vi "HandeEvents.vi"(0 "reference in":refnum<class "Logger.lvclass">, 11 "error in (no error)":errorcluster) -> (4 "reference out":refnum<class "Logger.lvclass">, 14 "dt":u32, 15 "error out":errorcluster)   [LabVIEW 2019, in "Logger.lvclass"]
uses:
  Logger.lvclass
  EventData.ctl
  EventCode.ctl
  Priority.ctl
  Logger.lvclass/Logger.ctl
  2f3f98d4-cfb0-4f81-b92a-0d178dd61f1e.vi
  1c0d0c3d-5d6b-42fa-8895-123650284108.vi
  DatabaseInterface_class/DatabaseInterface.lvclass
panel:
  out "remaining elements":T1[](array[typedef])
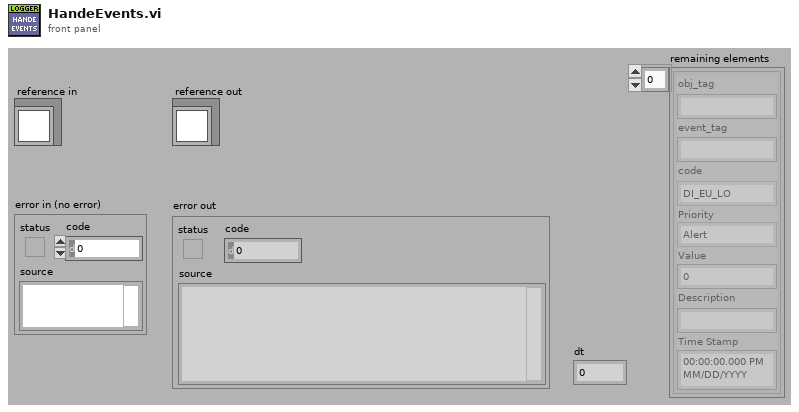
[diagram p1: front panel]
types:
  T1 = typedef "Logger.lvclass/EventData.ctl" = cluster{"obj_tag":string, "event_tag":string, "code":T2, "Priority":T3, "Value":dbl, "Description":string, "Time Stamp":timestamp}
  T2 = typedef "Logger.lvclass/EventCode.ctl" = enum16{"DI_EU_LO", "DI_EU_HI", "DIO_LO", "DIO_HI", "DI_RAW_LO", "DI_RAW_HI", "DO_LO", "DO_HI", "DA_OK", "DA_ALARM", "AA_HI", "AA_HIHI", "AA_LO", "AA_LOLO", "AA_OK", "CMD", "OUT_OF_RANGE_OK", "OUT_OF_RANGE_LO", "OUT_OF_RANGE_HI", "CONFIG", "DI_LO", "DI_HI"}
  T3 = typedef "Logger.lvclass/Priority.ctl" = enum16{"Alert", "Critical", "Error", "Warning", "Notice", "Informational", "Debug"}
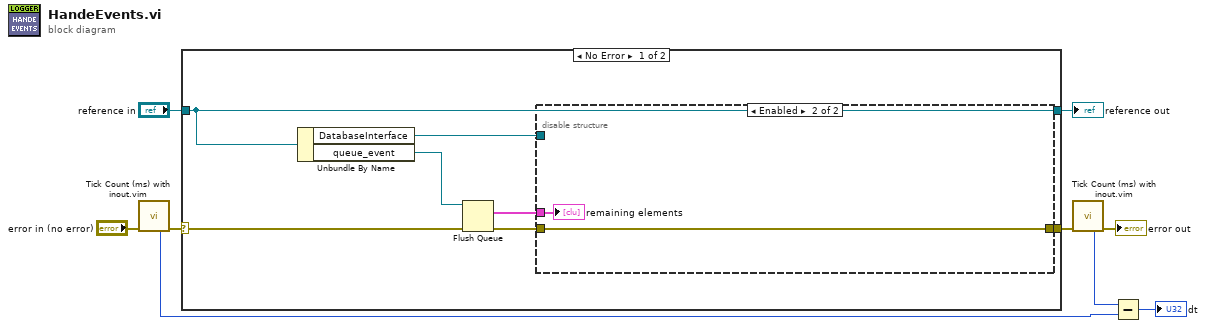
[diagram p0: block diagram]
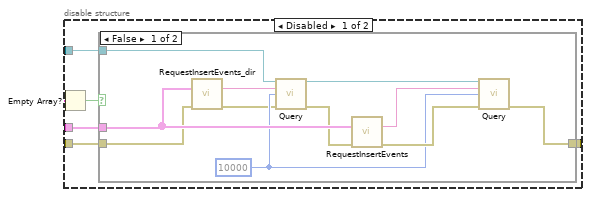
[diagram p2: hidden frame]
diagram:
  n1 = call "Tick Count (ms) with inout.vim"("in"="error in (no error)") -> ("millisecond timer value dub"=w4:u32, "out"=w7:errorcluster)  [unwired: 12 in, 1 out]
  n2 = case shown="No Error" w7 {
    selector: w7 -> [w16 w36]
    tunnel: [w15 w37] -> w2
    tunnel: "reference in" -> [w15 w37]
    tunnel: [w13 w36] -> w1
    frame No Error {
      n3 = Unbundle By Name(w15) -> ("DatabaseInterface"=w11:refnum<class "DatabaseInterface.lvclass">, "queue_event"=w14:refnum<queue>)
      n4 = Flush Queue(queue=w14, error in (no error)=w16) -> (remaining elements=w10:T1[], error out=w12:errorcluster)  [unwired: 1 out]
      n5 = disable-structure shown="Enabled" {
        disable-tunnel: [w21 w34] -> w13
        disable-tunnel: w12 -> [w20 w34]
        disable-tunnel: w11 -> [w19 _]
        disable-tunnel: w10 -> [w18 w35]
        frame Disabled {
          n6 = Empty Array?(array=w18) -> (empty?=w17:bool)
          n7 = case shown="False" w17 {
            tunnel: w18 -> [w32 _]
            tunnel: [w31 w33] -> w21
            tunnel: w20 -> [w30 w33]
            tunnel: w19 -> [w25 _]
            frame False {
              w26 = 10000 ("Timeout")
              n8 = call "RequestInsertEvents_dir.vi"("Events"=w32, "error in (no error)"=w30) -> ("request"=w27:string, "error out"=w23:errorcluster)  [unwired: 12 in]
              n9 = call-dynamic "Query.vi"("reference in"=w25, "Query"=w27, "Timeout"=w26, "error in (no error)"=w23) -> ("reference out"=w24:refnum<class "DatabaseInterface.lvclass">, "error out"=w22:errorcluster)  [unwired: 9 in, 1 out]
              n10 = call "RequestInsertEvents.vi"("Events"=w32, "error in (no error)"=w22) -> ("request"=w28:string, "error out"=w29:errorcluster)  [unwired: 12 in]
              n11 = call-dynamic "Query.vi"("reference in"=w24, "Query"=w28, "Timeout"=w26, "error in (no error)"=w29) -> ("error out"=w31:errorcluster)  [unwired: 9 in, 2 out]
            }
            frame True {
            }
          }
        }
        frame Enabled {
          "remaining elements" <- w35
        }
      }
    }
    frame Error {
    }
  }
  "reference out" <- w2
  n12 = call "Tick Count (ms) with inout.vim"("in"=w1) -> ("millisecond timer value dub"=w5:u32, "out"=→"error out":errorcluster)  [unwired: 12 in, 1 out]
  n13 = Subtract(x=w5, y=w4) -> (x-y=→"dt":u32)
